vi "generate wave packet V2.vi"(7 "number of grid points":i32=300, 8 "complex region":T2={"max re"=5.161869466666667e-06, "min re"=5.176843333333334e-06, "max im"=-2.467216e-05, "min im"=-0.001573233, "delta re"=0.003211203, "delta im"=0.00165815, "center re"=0.0015485608400000002, "delta  z"=0.0015530530000000002+0.0i, "center im"=0.0, "center z"=0.0+0.0i, "d im"=0.0, "d re"=0.0, "d z"=0.0+0.0i}, 11 "wavepacket in":T1={"R"=0.5, "wave number"=22.0, "delta k"=7.0, "radii vector"=[], "radial section"=[], "wave vector"=22.0, "wavepacket is"=TRUE} {"delta k" format="%#_3f"; "wave number" format="%#_3f"; "R" format="%#_3f"}) -> (1 "pond array out":cdb[][](array[numeric]), 2 "wavepacket array out":cdb[][](array[numeric]), 3 "wavepacket out":T1={"R"=0.5, "wave number"=22.0, "delta k"=7.0, "radii vector"=[], "radial section"=[], "wave vector"=22.0, "wavepacket is"=TRUE} {"delta k" format="%#_3f"; "wave number" format="%#_3f"; "R" format="%#_3f"})   [LabVIEW 2021]
uses:
  complex region.ctl
  wavepacket.ctl
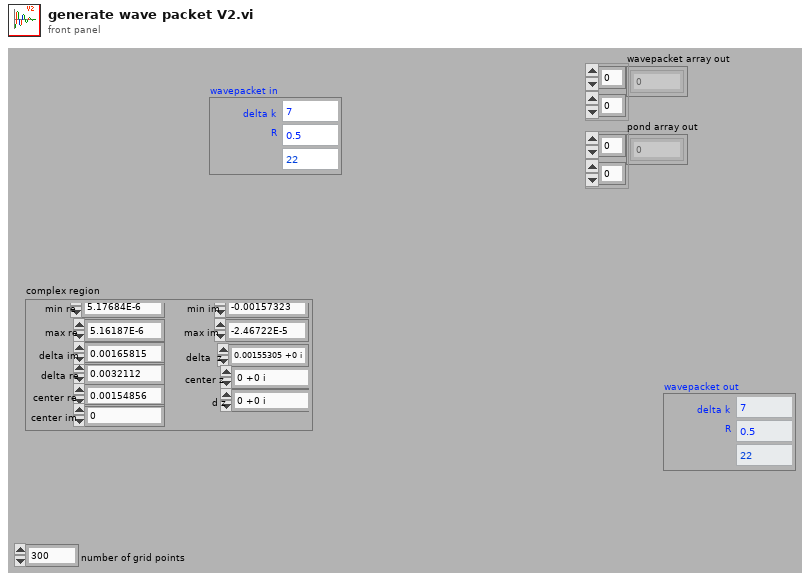
[diagram p1: front panel]
types:
  T1 = typedef "wavepacket.ctl" = cluster{"R":dbl, "wave number":dbl, "delta k":dbl, "radii vector":dbl[], "radial section":cdb[], "wave vector":dbl, "wavepacket is":bool}
  T2 = typedef "complex region.ctl" = cluster{"max re":dbl, "min re":dbl, "max im":dbl, "min im":dbl, "delta re":dbl, "delta im":dbl, "center re":dbl, "delta  z":cdb, "center im":dbl, "center z":cdb, "d im":dbl, "d re":dbl, "d z":cdb}
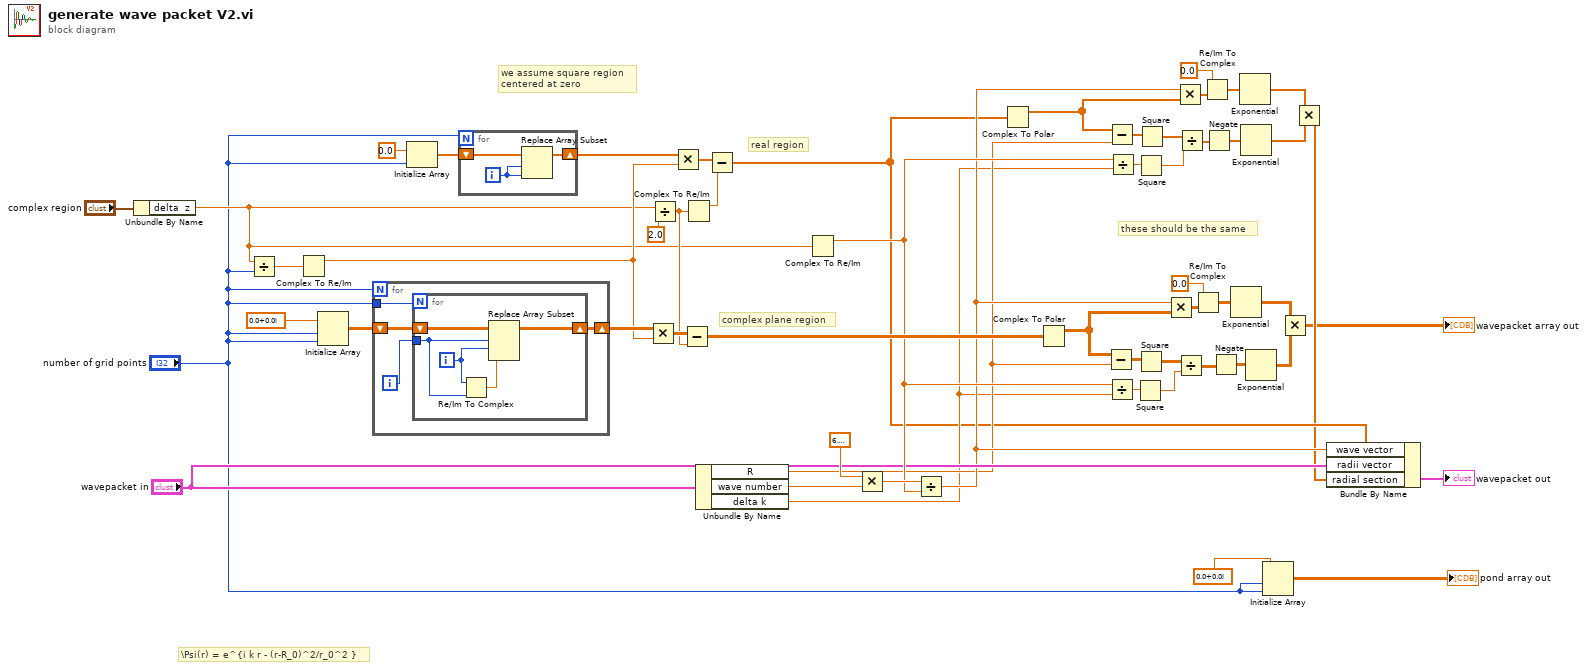
[diagram p0: block diagram]
diagram:
  # "complex plane region"
  # "real region"
  # "we assume square region\ncentered at zero"
  # "\\Psi(r) = e^{i k r - (r-R_0)^2/r_0^2 }"
  # "these should be the same"
  n1 = Unbundle By Name("complex region") -> ("delta  z"=w14:cdb)
  n2 = Divide(x=w14, y="number of grid points") -> (x/y=w24:cdb)
  n3 = Complex To Re/Im(x + iy=w24) -> (x=w21:dbl)  [unwired: 1 out]
  n4 = Initialize Array(cdb 0.0+0.0i ("element"), "number of grid points", "number of grid points") -> (w27:cdb[][])
  n5 = for {
    N: "number of grid points" -> [_]
    tunnel: "number of grid points" -> [w58]
    shift-right: [w57] -> w22
    shift-left: w27 -> [w59]
    i -> [w56]
    n6 = for {
      N: w58 -> [_]
      shift-right: [w63] -> w57
      shift-left: w59 -> [w64]
      tunnel: w56 -> [w60]
      i -> [w61]
      n7 = Re/Im To Complex(1:w60, 2:w61) -> (0:w62:cdb)
      n8 = Replace Array Subset(array=w64, new element=w62, index (row)=w60, index (col)=w61) -> (w63:cdb[][])
    }
  }
  n9 = Initialize Array(0.0 ("element"), "number of grid points") -> (w32:dbl[])
  n10 = for {
    N: "number of grid points" -> [_]
    shift-right: [w66] -> w30
    shift-left: w32 -> [w67]
    i -> [w65]
    n11 = Replace Array Subset(array=w67, new element=w65, index=w65) -> (w66:dbl[])
  }
  n12 = Multiply(x=w22, y=w21) -> (x*y=w26:cdb[][])
  n13 = Divide(x=w14, y=2.0) -> (x/y=w23:cdb)
  n14 = Multiply(x=w30, y=w21) -> (x*y=w29:dbl[])
  n15 = Subtract(x=w26, y=w23) -> (x-y=w20:cdb[][])
  n16 = Complex To Re/Im(x + iy=w23) -> (x=w25:dbl)  [unwired: 1 out]
  n17 = Unbundle By Name("wavepacket in") -> ("R"=w9:dbl, "wave number"=w11:dbl, "delta k"=w8:dbl)
  n18 = Subtract(x=w29, y=w25) -> (x-y=w7:dbl[])
  n19 = Complex To Re/Im(x + iy=w14) -> (x=w13:dbl)  [unwired: 1 out]
  n20 = Multiply(x=6.283185307179586, y=w11) -> (x*y=w45:dbl)
  n21 = Divide(x=w45, y=w13) -> (x/y=w10:dbl)
  n22 = Complex To Polar(r * e^(i*theta)=w7) -> (r=w36:dbl[])  [unwired: 1 out]
  n23 = Complex To Polar(r * e^(i*theta)=w20) -> (r=w15:dbl[][])  [unwired: 1 out]
  n24 = Subtract(x=w15, y=w9) -> (x-y=w53:dbl[][])
  n25 = Subtract(x=w36, y=w9) -> (x-y=w43:dbl[])
  n26 = Divide(x=w13, y=w8) -> (x/y=w52:dbl)
  n27 = Divide(x=w13, y=w8) -> (x/y=w42:dbl)
  n28 = Square(x=w52) -> (x^2=w34:dbl)
  n29 = Square(x=w42) -> (x^2=w35:dbl)
  n30 = Square(x=w53) -> (x^2=w54:dbl[][])
  n31 = Square(x=w43) -> (x^2=w44:dbl[])
  n32 = Multiply(x=w10, y=w15) -> (x*y=w51:dbl[][])
  n33 = Multiply(x=w10, y=w36) -> (x*y=w41:dbl[])
  n34 = Divide(x=w54, y=w34) -> (x/y=w17:dbl[][])
  n35 = Divide(x=w44, y=w35) -> (x/y=w19:dbl[])
  n36 = Re/Im To Complex(1:w51, 2:0.0 ("x")) -> (0:w49:cdb[][])
  n37 = Re/Im To Complex(1:w41, 2:0.0 ("x")) -> (0:w39:cdb[])
  n38 = Negate(x=w19) -> (-x=w18:dbl[])
  n39 = Negate(x=w17) -> (-x=w16:dbl[][])
  n40 = Exponential(1:w49) -> (0:w47:cdb[][])
  n41 = Exponential(1:w39) -> (0:w37:cdb[])
  n42 = Exponential(1:w18) -> (0:w38:dbl[])
  n43 = Exponential(1:w16) -> (0:w48:dbl[][])
  n44 = Initialize Array(cdb 0.0+0.0i ("element"), "number of grid points", "number of grid points") -> (→"pond array out":cdb[][])
  n45 = Multiply(x=w48, y=w47) -> (x*y=→"wavepacket array out":cdb[][])
  n46 = Multiply(x=w38, y=w37) -> (x*y=w6:cdb[])
  n47 = Bundle By Name(cluster="wavepacket in", "wave vector"=w10, "radii vector"=w7, "radial section"=w6) -> (→"wavepacket out":T1)
